vi "FdxCmdTxStaticRegsControlCvi.vi"(8 "error in":errorcluster, 9 "TxStaticRegs":T1, 11 "InstrumentHandle_port":u32) -> (0 "error out":errorcluster, 3 "InstrumentHandle_port":u32)   [LabVIEW 2020, in "AIM664LV.lvlib"]
doc: "This function is used to setup the Static Transmit Registers of a port. This is especially used in Generic Transmit Mode, together with corresponding Payload Generation Modes (see AiFdxCmdTxQueueWrite command). For other Transmit Modes (Replay and Individual) this command has no effect."
uses:
  AIM664LV.lvlib
  AFDX_LibraryAdmin/FdxGlobalDllPath.vi
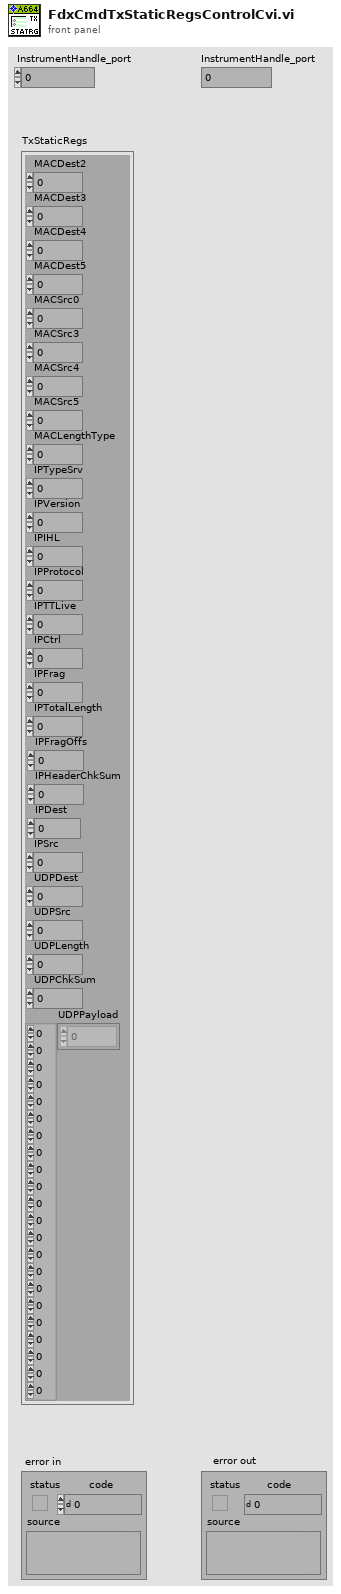
[diagram p1: front panel]
types:
  T1 = cluster{"MACDest2":u8, "MACDest3":u8, "MACDest4":u8, "MACDest5":u8, "MACSrc0":u8, "MACSrc3":u8, "MACSrc4":u8, "MACSrc5":u8, "MACLengthType":u16, "IPTypeSrv":u8, "IPVersion":u8, "IPIHL":u8, "IPProtocol":u8, "IPTTLive":u8, "IPCtrl":u8, "IPFrag":u16, "IPTotalLength":u16, "IPFragOffs":u16, "IPHeaderChkSum":u16, "IPDest":u32, "IPSrc":u32, "UDPDest":u16, "UDPSrc":u16, "UDPLength":u16, "UDPChkSum":u16, "UDPPayload":u8[][][][][][][][][][][][][][][][][][][][][][]}
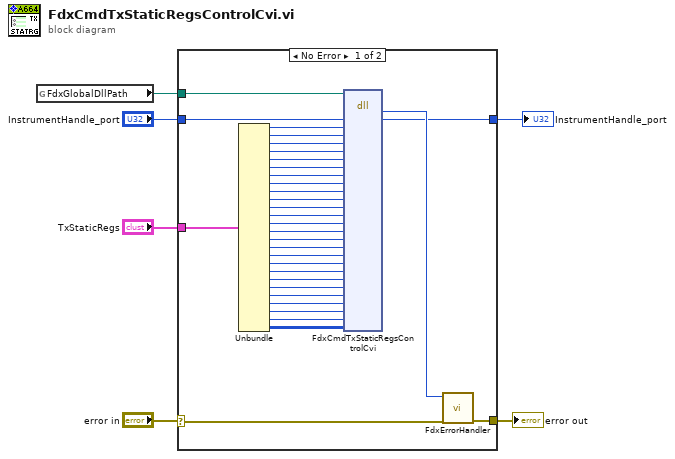
[diagram p0: block diagram]
diagram:
  n1 = global read "FdxGlobalDllPath.vi" "FdxGlobalDllPath"() -> (w4:path)
  n2 = case shown="No Error" "error in" {
    selector: "error in" -> [w38 w41]
    tunnel: [w39 w41] -> w6
    tunnel: w4 -> [w10 _]
    tunnel: "InstrumentHandle_port" -> [w9 w40]
    tunnel: [w8 w40] -> w2
    tunnel: "TxStaticRegs" -> [w7 _]
    frame No Error {
      n3 = Unbundle(w7) -> ("MACDest2"=w36:u8, "MACDest3"=w35:u8, "MACDest4"=w34:u8, "MACDest5"=w33:u8, "MACSrc0"=w32:u8, "MACSrc3"=w31:u8, "MACSrc4"=w30:u8, "MACSrc5"=w26:u8, "MACLengthType"=w29:u16, "IPTypeSrv"=w28:u8, "IPVersion"=w27:u8, "IPIHL"=w25:u8, "IPProtocol"=w24:u8, "IPTTLive"=w23:u8, "IPCtrl"=w22:u8, "IPFrag"=w21:u16, "IPTotalLength"=w20:u16, "IPFragOffs"=w19:u16, "IPHeaderChkSum"=w18:u16, "IPDest"=w17:u32, "IPSrc"=w16:u32, "UDPDest"=w15:u16, "UDPSrc"=w14:u16, "UDPLength"=w13:u16, "UDPChkSum"=w12:u16, "UDPPayload"=w11:u8[][][][][][][][][][][][][][][][][][][][][][])
      n4 = dll-call lib="aim_fdx.19.dll" fn="FdxCmdTxStaticRegsControlCvi"(path in=w10, "InstrumentHandle"=w9, "MACDest2"=w36, "MACDest3"=w35, "MACDest4"=w34, "MACDest5"=w33, "MACSrc0"=w32, "MACSrc3"=w31, "MACSrc4"=w30, "MACSrc5"=w26, "MACLengthType"=w29, "IPTypeSrv"=w28, "IPVersion"=w27, "IPIHL"=w25, "IPProtocol"=w24, "IPTTLive"=w23, "IPCtrl"=w22, "IPFrag"=w21, "IPTotalLength"=w20, "IPFragOffs"=w19, "IPHeaderChkSum"=w18, "IPDest"=w17, "IPSrc"=w16, "UDPDest"=w15, "UDPSrc"=w14, "UDPLength"=w13, "UDPChkSum"=w12, "UDPPayload"=w11) -> ("status"=w37:i32, "InstrumentHandle"=w8:u32)  [unwired: 28 in, 2 out]
      n5 = call "FdxErrorHandler.vi"("error in"=w38, "AIM Error"=w37) -> ("error out"=w39:errorcluster)  [unwired: 9 in]
    }
    frame Error {
    }
  }
  "error out" <- w6
  "InstrumentHandle_port" <- w2
